vi "AFS Calculatte_Percentage.vi"(6 "Delta C":string[](array[string]), 8 "Error In":errorcluster, 9 "Target Cap (fF)":dbl) -> (0 "Error Out":errorcluster, 4 "% Detla C":string[](array[string]))   [LabVIEW 2017]
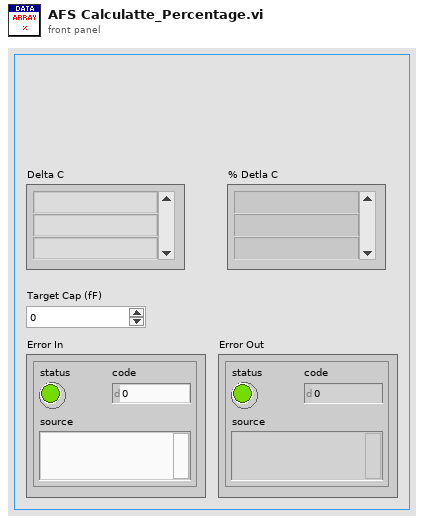
[diagram p1: front panel]
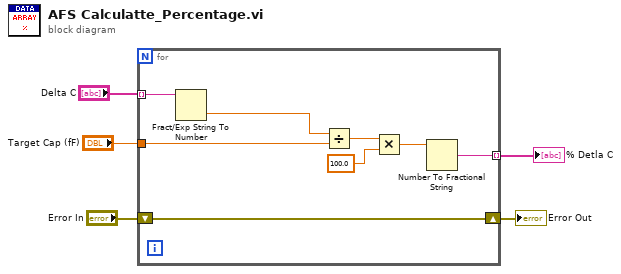
[diagram p0: block diagram]
diagram:
  n1 = for {
    tunnel: "Delta C" -> [w13] mode=indexing
    tunnel: "Target Cap (fF)" -> [w12]
    tunnel: [w11] -> w3 mode=indexing
    shift-right: [w7] -> w1
    shift-left: "Error In" -> [w7]
    n2 = Fract/Exp String To Number(string=w13) -> (number=w6:dbl)  [unwired: 3 in, 1 out]
    n3 = Divide(x=w6, y=w12) -> (x/y=w9:dbl)
    n4 = Multiply(x=w9, y=100.0) -> (x*y=w10:dbl)
    n5 = Number To Fractional String(number=w10) -> (F-format string=w11:string)  [unwired: 3 in]
  }
  "Error Out" <- w1
  "% Detla C" <- w3
